vi "Delete Dvr.vi"(8 "Error In":errorcluster, 10 "Data Value Reference":refnum<data-value>) -> (0 "Error Out":errorcluster)   [LabVIEW 2021, in "Calculator.lvlib" / "NumericOperation.lvclass"]
doc: "This VI deletes the Data Value Reference."
uses:
  NumericOperation.lvclass
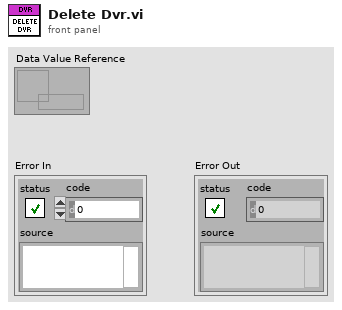
[diagram p1: front panel]
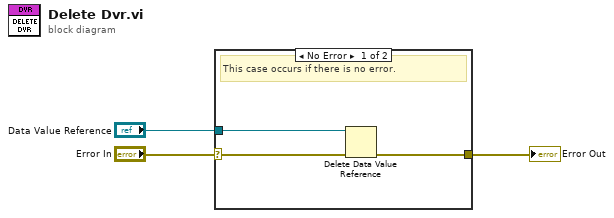
[diagram p0: block diagram]
diagram:
  n1 = case shown="No Error" "Error In" {
    selector: "Error In" -> [w5 w7]
    tunnel: [w4 w7] -> w2
    tunnel: "Data Value Reference" -> [w6 _]
    frame No Error {
      # "This case occurs if there is no error."
      n2 = Delete Data Value Reference(data value reference=w6, error in=w5) -> (error out=w4:errorcluster)  [unwired: 1 out]
    }
    frame Error {
      # "This case occurs if there is any error."
    }
  }
  "Error Out" <- w2
